vi "LimitCurrent.vi"(5 "Battle Short":bool, 6 "Error In":errorcluster, 8 "Current In":dbl, 9 "Current Limit Parameters":T1 {"Min Cell Voltage Actual Value" format="%#.2f"; "Max Cell Voltage Actual Value" format="%#.2f"}) -> (0 "Error Out":errorcluster, 2 "Current Out":dbl, 3 "Limited?":bool=TRUE)   [LabVIEW 2014]
uses:
  <userlib>/cRIO Master Files/Controls/CurrentLimitParameters.ctl
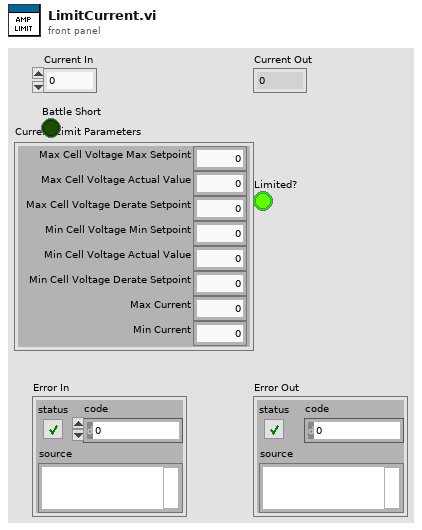
[diagram p1: front panel]
types:
  T1 = typedef "CurrentLimitParameters.ctl" = cluster{"Max Cell Voltage Max Setpoint":dbl, "Max Cell Voltage Actual Value":dbl, "Max Cell Voltage Derate Setpoint":dbl, "Min Cell Voltage Min Setpoint":dbl, "Min Cell Voltage Actual Value":dbl, "Min Cell Voltage Derate Setpoint":dbl, "Max Current":dbl, "Min Current":dbl}
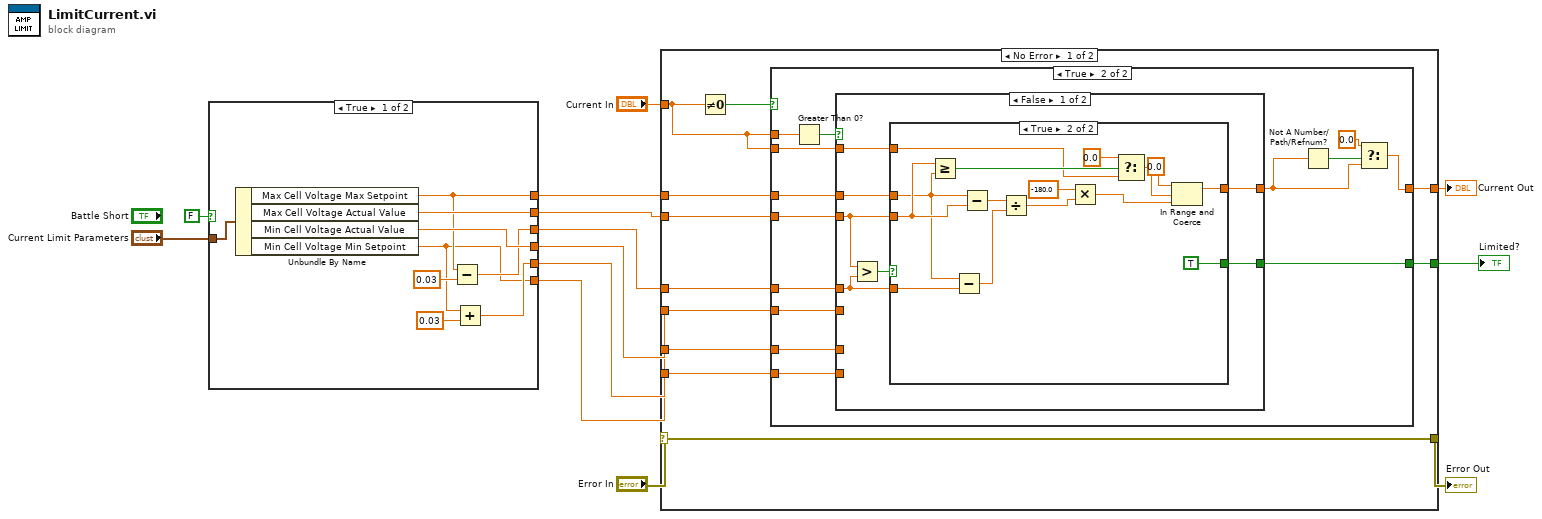
[diagram p0: block diagram]
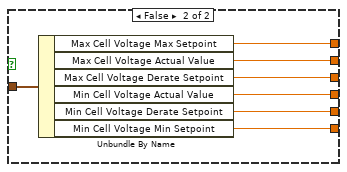
[diagram p2: hidden frame]
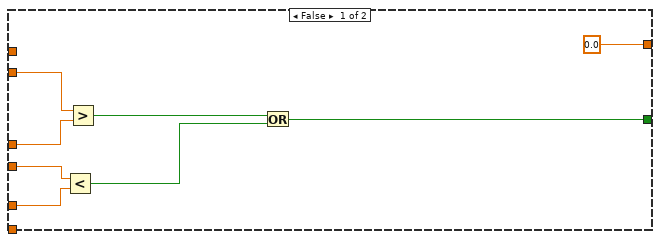
[diagram p3: hidden frame]
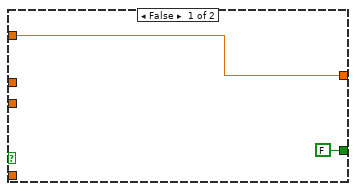
[diagram p4: hidden frame]
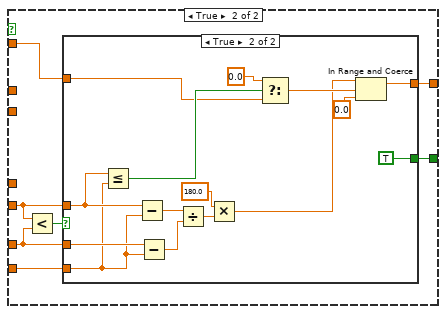
[diagram p5: hidden frame]
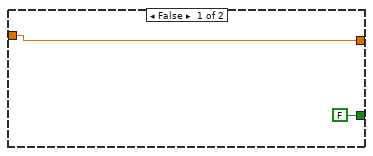
[diagram p6: hidden frame]
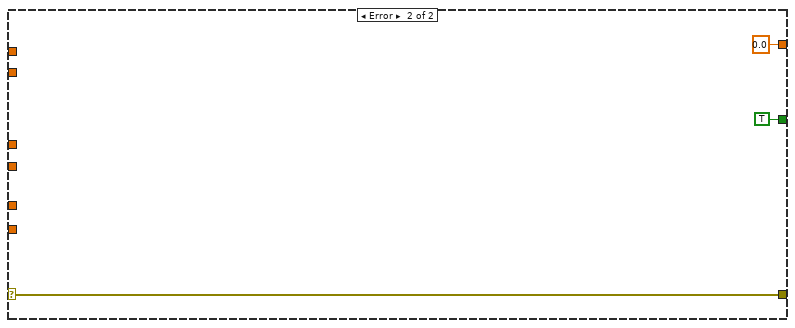
[diagram p7: hidden frame]
diagram:
  n1 = case shown="True" FALSE {
    tunnel: [w18 w29] -> w8
    tunnel: [w21 w28] -> w7
    tunnel: [w17 w27] -> w6
    tunnel: [w20 w26] -> w5
    tunnel: [w15 w25] -> w4
    tunnel: [w14 w24] -> w3
    tunnel: "Current Limit Parameters" -> [w22 w23]
    frame True {
      n2 = Unbundle By Name(w22) -> ("Max Cell Voltage Max Setpoint"=w18:dbl, "Max Cell Voltage Actual Value"=w21:dbl, "Min Cell Voltage Actual Value"=w20:dbl, "Min Cell Voltage Min Setpoint"=w14:dbl)
      n3 = Subtract(x=w18, y=0.03) -> (x-y=w17:dbl)
      n4 = Add(x=w14, y=0.03) -> (x+y=w15:dbl)
    }
    frame False {
      n5 = Unbundle By Name(w23) -> ("Max Cell Voltage Max Setpoint"=w29:dbl, "Max Cell Voltage Actual Value"=w28:dbl, "Max Cell Voltage Derate Setpoint"=w27:dbl, "Min Cell Voltage Actual Value"=w26:dbl, "Min Cell Voltage Derate Setpoint"=w25:dbl, "Min Cell Voltage Min Setpoint"=w24:dbl)
    }
  }
  n6 = case shown="No Error" "Error In" {
    selector: "Error In" -> [w31 w113]
    tunnel: [w39 0.0 ("t")] -> w13
    tunnel: w7 -> [w38 _]
    tunnel: w6 -> [w37 _]
    tunnel: "Current In" -> [w36 _]
    tunnel: w8 -> [w35 _]
    tunnel: w3 -> [w34 _]
    tunnel: w5 -> [w33 _]
    tunnel: w4 -> [w32 _]
    tunnel: [w31 w113] -> w10
    tunnel: [w30 TRUE] -> w9
    frame No Error {
      n7 = Not Equal To 0?(x=w36) -> (x != 0?=w40:bool)
      n8 = case shown="True" w40 {
        tunnel: [0.0 w52] -> w39
        tunnel: w36 -> [_ w62]
        tunnel: w38 -> [w43 w60]
        tunnel: w37 -> [w42 w59]
        tunnel: w36 -> [_ w58]
        tunnel: w35 -> [_ w57]
        tunnel: w34 -> [_ w56]
        tunnel: w33 -> [w46 w55]
        tunnel: w32 -> [w45 w54]
        tunnel: [w44 w49] -> w30
        frame False {
          n9 = Less?(x=w46, y=w45) -> (x < y?=w47:bool)
          n10 = Greater?(x=w43, y=w42) -> (0:w41:bool)
          n11 = Or(x=w41, y=w47) -> (x .or. y?=w44:bool)
        }
        frame True {
          n12 = Greater Than 0?(x=w62) -> (x > 0?=w61:bool)
          n13 = case shown="False" w61 {
            tunnel: w60 -> [w66 _]
            tunnel: w59 -> [w65 _]
            tunnel: w58 -> [w69 w89]
            tunnel: [w67 w88] -> w51
            tunnel: w57 -> [w64 _]
            tunnel: w56 -> [_ w90]
            tunnel: w55 -> [_ w92]
            tunnel: w54 -> [_ w91]
            tunnel: [w63 w87] -> w49
            frame False {
              n14 = Greater?(x=w66, y=w65) -> (0:w68:bool)
              n15 = case shown="True" w68 {
                tunnel: w69 -> [w71 w75]
                tunnel: [w71 w80] -> w67
                tunnel: w66 -> [_ w82]
                tunnel: w65 -> [_ w85]
                tunnel: w64 -> [_ w81]
                tunnel: [FALSE TRUE] -> w63
                frame False {
                }
                frame True {
                  n16 = Greater Or Equal?(x=w82, y=w81) -> (x >= y?=w77:bool)
                  n17 = Subtract(x=w81, y=w85) -> (x-y=w84:dbl)
                  n18 = Subtract(x=w81, y=w82) -> (x-y=w86:dbl)
                  n19 = Divide(x=w86, y=w84) -> (x/y=w83:dbl)
                  n20 = Multiply(x=-180.0, y=w83) -> (x*y=w73:dbl)
                  n21 = Select(t=0.0, s=w77, f=w75) -> (s? t:f=w78:dbl)
                  n22 = In Range and Coerce(upper limit=0.0 ("lower limit"), x=w78, lower limit=w73) -> (coerced(x)=w80:dbl)  [unwired: 1 out]
                }
              }
            }
            frame True {
              n23 = Less?(x=w92, y=w91) -> (x < y?=w93:bool)
              n24 = case shown="True" w93 {
                tunnel: w92 -> [_ w106]
                tunnel: w91 -> [_ w109]
                tunnel: w90 -> [_ w105]
                tunnel: w89 -> [w95 w99]
                tunnel: [w95 w102] -> w88
                tunnel: [FALSE TRUE] -> w87
                frame False {
                }
                frame True {
                  n25 = Less Or Equal?(x=w106, y=w105) -> (x <= y?=w104:bool)
                  n26 = Subtract(x=w106, y=w105) -> (x-y=w110:dbl)
                  n27 = Subtract(x=w109, y=w105) -> (x-y=w108:dbl)
                  n28 = Divide(x=w110, y=w108) -> (x/y=w107:dbl)
                  n29 = Multiply(x=180.0, y=w107) -> (x*y=w98:dbl)
                  n30 = Select(t=0.0, s=w104, f=w99) -> (s? t:f=w101:dbl)
                  n31 = In Range and Coerce(upper limit=w98, x=w101, lower limit=0.0 ("upper limit")) -> (coerced(x)=w102:dbl)  [unwired: 1 out]
                }
              }
            }
          }
          n32 = Not A Number/Path/Refnum?(number/path/refnum=w51) -> (NaN/Path/Refnum?=w50:bool)
          n33 = Select(t=0.0, s=w50, f=w51) -> (s? t:f=w52:dbl)
        }
      }
    }
    frame Error {
    }
  }
  "Current Out" <- w13
  "Error Out" <- w10
  "Limited?" <- w9
